vi "GraphWidthAndLegendVisible(SubVI).vi"(7 "Arr Refnum":refnum<vi>, 8 "Error In":errorcluster, 9 "This VI":refnum<vi>, 10 "XYGraph Refnum":refnum<vi>, 11 "Legend":refnum<vi>) -> (0 "Error Out":errorcluster)   [LabVIEW 2018]
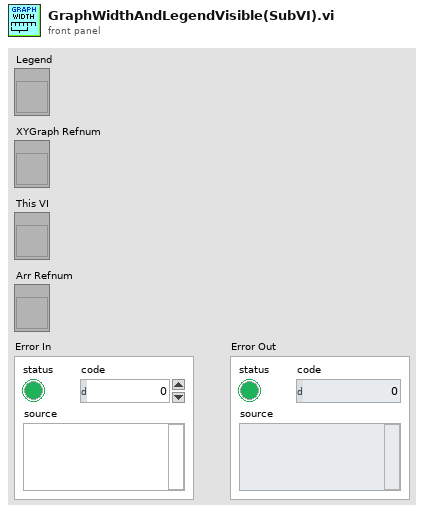
[diagram p1: front panel]
types:
  T1 = typedef "LVRectTypeDef.ctl" = cluster{"Left":i16, "Top":i16, "Right":i16, "Bottom":i16}
  T2 = typedef "Line.ctl" = cluster{"Width":dbl, "Color":i64, "Array Oy":dbl[], "Array Ox":dbl[], "Name":string, "Plot Visible":T3}
  T3 = typedef "View.ctl" = bool
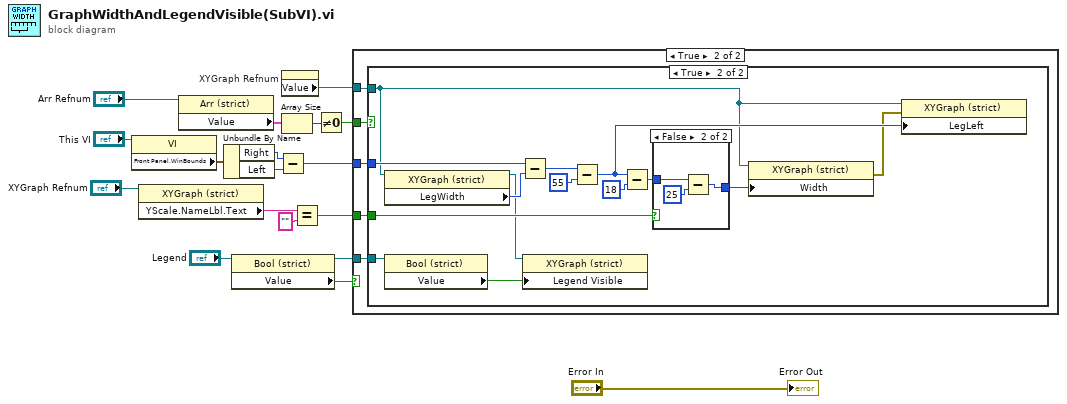
[diagram p0: block diagram]
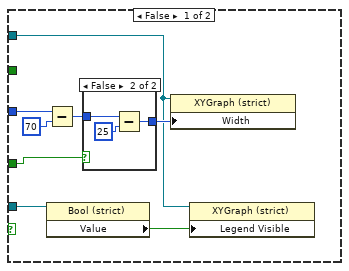
[diagram p2: hidden frame]
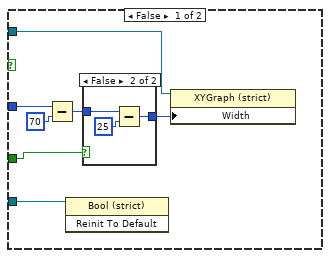
[diagram p4: hidden frame]
diagram:
  n1 = property class="VI"(reference="This VI") -> ("Front Panel.WinBounds"=w11:T1)  [unwired: 1 in, 2 out]
  n2 = property on="Property Node" class="XYGraph (strict)"(reference="XYGraph Refnum") -> ("YScale.NameLbl.Text"=w4:string)  [unwired: 1 in, 2 out]
  n3 = property on="Property Node" class="Arr (strict)"(reference="Arr Refnum") -> ("Value"=w7:T2[])  [unwired: 1 in, 2 out]
  n4 = Unbundle By Name(w11) -> ("Right"=w9:i16, "Left"=w1:i16)
  n5 = property on="Property Node" class="Bool (strict)"(reference="Legend") -> (reference out=w16:refnum<vi>, "Value"=w12:bool)  [unwired: 1 in, 1 out]
  n6 = Subtract(x=w9, y=w1) -> (x-y=w3:i16)
  n7 = property on="XYGraph Refnum" class="LVObjRef (strict)"() -> ("Value"=w17:refnum<vi>)  [unwired: 2 in, 2 out]
  n8 = Array Size(array=w7) -> (size(s)=w8:i32)
  n9 = Equal?(x=w4, y="") -> (x = y?=w2:bool)
  n10 = Not Equal To 0?(x=w8) -> (x != 0?=w6:bool)
  n11 = case shown="True" w12 {
    tunnel: w3 -> [w19 w35]
    tunnel: w6 -> [_ w34]
    tunnel: w16 -> [w25 w32]
    tunnel: w17 -> [w20 w33]
    tunnel: w2 -> [w21 w31]
    frame False {
      n12 = Subtract(x=w19, y=u32 70) -> (x-y=w24:u32)
      n13 = property on="Property Node" class="Bool (strict)"(reference=w25) -> ("Value"=w26:bool)  [unwired: 1 in, 2 out]
      n14 = case shown="False" w21 {
        tunnel: w24 -> [w27 w30]
        tunnel: [w27 w28] -> w23
        frame True {
        }
        frame False {
          n15 = Subtract(x=w30, y=25) -> (x-y=w28:u32)
        }
      }
      n16 = property on="Property Node" class="XYGraph (strict)"(reference=w20, "Width"=w23) -> ()  [unwired: 1 in, 2 out]
      n17 = property on="Property Node" class="XYGraph (strict)"(reference=w20, "Legend Visible"=w26) -> ()  [unwired: 1 in, 2 out]
    }
    frame True {
      n18 = case shown="True" w34 {
        tunnel: w35 -> [w36 w58]
        tunnel: w33 -> [w37 w48]
        tunnel: w32 -> [w42 w59]
        tunnel: w31 -> [w38 w53]
        frame False {
          n19 = Subtract(x=w36, y=u32 70) -> (x-y=w41:u32)
          n20 = invoke on="Invoke Node" class="Bool (strict)" method="Reinit To Default"(reference=w42) -> ()  [unwired: 2 in, 3 out]
          n21 = case shown="False" w38 {
            tunnel: w41 -> [w43 w46]
            tunnel: [w43 w44] -> w40
            frame True {
            }
            frame False {
              n22 = Subtract(x=w46, y=25) -> (x-y=w44:u32)
            }
          }
          n23 = property on="Property Node" class="XYGraph (strict)"(reference=w37, "Width"=w40) -> ()  [unwired: 1 in, 2 out]
        }
        frame True {
          n24 = property on="Property Node" class="XYGraph (strict)"(reference=w48) -> (reference out=w47:refnum<vi>, "LegWidth"=w57:u32)  [unwired: 1 in, 1 out]
          n25 = property on="Property Node" class="Bool (strict)"(reference=w59) -> ("Value"=w60:bool)  [unwired: 1 in, 2 out]
          n26 = Subtract(x=w58, y=w57) -> (x-y=w54:u32)
          n27 = property on="Property Node" class="XYGraph (strict)"(reference=w47, "Legend Visible"=w60) -> ()  [unwired: 1 in, 2 out]
          n28 = Subtract(x=w54, y=u32 55) -> (x-y=w50:u32)
          n29 = Subtract(x=w50, y=u32 18) -> (x-y=w52:u32)
          n30 = case shown="False" w53 {
            tunnel: w52 -> [w61 w64]
            tunnel: [w61 w62] -> w51
            frame True {
            }
            frame False {
              n31 = Subtract(x=w64, y=25) -> (x-y=w62:u32)
            }
          }
          n32 = property on="Property Node" class="XYGraph (strict)"(reference=w48, "Width"=w51) -> (error out=w49:errorcluster)  [unwired: 1 in, 1 out]
          n33 = property on="Property Node" class="XYGraph (strict)"(reference=w48, error in=w49, "LegLeft"=w50) -> ()  [unwired: 2 out]
        }
      }
    }
  }
  "Error Out" <- "Error In"
